vi "testcase - temp to permanent.vi"   [LabVIEW 2017]
uses:
  INI-Static-Variable-Support/INI-Static-Variable-Support.lvlib
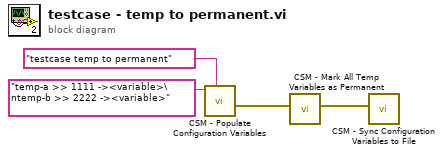
[diagram p0: block diagram]
diagram:
  n1 = call "CSM - Populate Configuration Variables.vi"("Section Name(\"\" as Default)"="testcase temp to permanent" ("Section Name(\"\" as Default)"), "String in"="temp-a >> 1111 -><variable>\ntemp-b >> 2222 -><variable>") -> ("error out"=w3:errorcluster)  [unwired: 6 in, 1 out]
  n2 = call "CSM - Mark All Temp Variables as Permanent.vi"("error in (no error)"=w3) -> ("error out"=w2:errorcluster)  [unwired: 8 in]
  n3 = call "CSM - Sync Configuration Variables to File.vi"("error in (no error)"=w2) -> ()  [unwired: 8 in, 1 out]
